vi "genImageMatrix.vi"(6 "Orientation":bool, 8 "Phase":dbl, 9 "Cycles":dbl, 10 "Y resolution":i32, 11 "X Resolution":i32) -> (1 "genSize":i32[](array[numeric]), 3 "Scan Image":u8[][](array[numeric]))   [LabVIEW 2017]
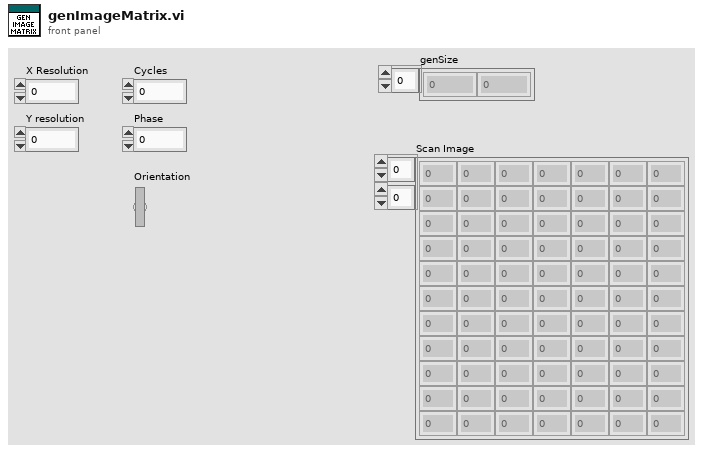
[diagram p1: front panel]
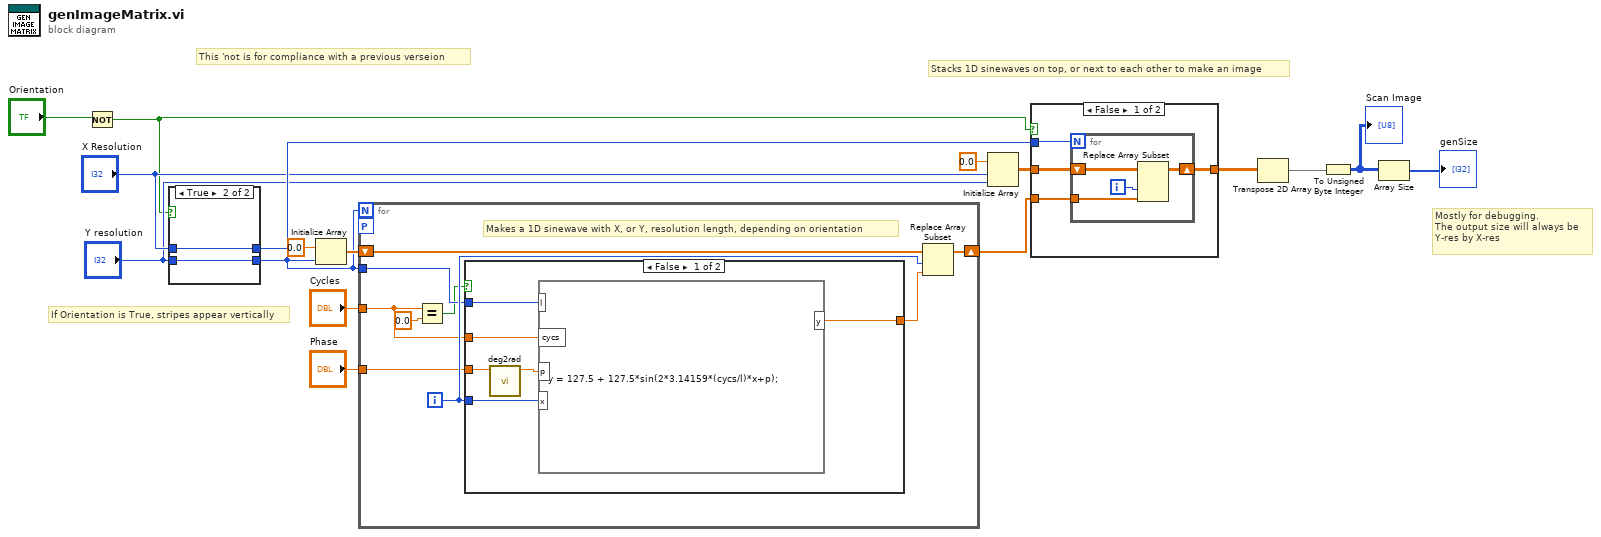
[diagram p0: block diagram]
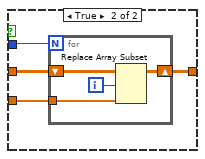
[diagram p2: hidden frame]
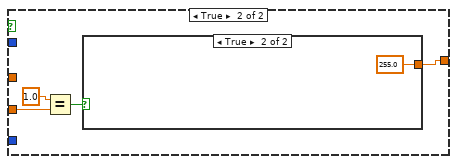
[diagram p4: hidden frame]
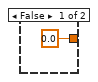
[diagram p5: hidden frame]
diagram:
  # "This 'not is for compliance with a previous verseion"
  # "Mostly for debugging.\nThe output size will always be\nY-res by X-res"
  # "Stacks 1D sinewaves on top, or next to each other to make an image"
  # "If Orientation is True, stripes appear vertically"
  n1 = Not(x="Orientation") -> (.not. x?=w1:bool)
  n2 = case shown="True" w1 {
    tunnel: [w18 w20] -> w9
    tunnel: "Y resolution" -> [w19 w20]
    tunnel: "X Resolution" -> [w18 w21]
    tunnel: [w19 w21] -> w7
    frame False {
    }
    frame True {
    }
  }
  n3 = Initialize Array(0.0 ("element"), w9) -> (w15:dbl[])
  n4 = for {
    N: w9 -> [_]
    shift-right: [w28] -> w8
    shift-left: w15 -> [w29]
    tunnel: "Cycles" -> [w22]
    tunnel: "Phase" -> [w26]
    tunnel: w9 -> [w25]
    workers-P: _ -> [_]
    i -> [w27]
    # "Makes a 1D sinewave with X, or Y, resolution length, depending on orientation"
    n5 = Equal?(x=w22, y=0.0) -> (x = y?=w24:bool)
    n6 = case shown="False" w24 {
      tunnel: [w36 w37] -> w30
      tunnel: w27 -> [w35 _]
      tunnel: w22 -> [w34 _]
      tunnel: w26 -> [w32 w40]
      tunnel: w25 -> [w33 _]
      frame False {
        n7 = call "deg2rad.vi"("Degrees"=w32) -> ("Radians"=w31:dbl)  [unwired: 10 in]
        n8 = formula code="y = 127.5 + 127.5*sin(2*3.14159*(cycs/l)*x+p);"("l"=w33, "cycs"=w34, "p"=w31, "x"=w35) -> ("y"=w36:dbl)
      }
      frame True {
        n9 = Equal?(x=1.0, y=w40) -> (x = y?=w38:bool)
        n10 = case shown="True" w38 {
          tunnel: [0.0 255.0] -> w37
          frame False {
          }
          frame True {
          }
        }
      }
    }
    n11 = Replace Array Subset(array=w29, new element=w30, index=w27) -> (w28:dbl[])
  }
  n12 = Initialize Array(0.0 ("element"), "X Resolution", "Y resolution") -> (w14:dbl[][])
  n13 = case shown="False" w1 {
    tunnel: w14 -> [w45 w54]
    tunnel: w8 -> [w44 w53]
    tunnel: [w43 w52] -> w4
    tunnel: w7 -> [w46 w51]
    frame False {
      n14 = for {
        N: w46 -> [_]
        shift-right: [w49] -> w43
        shift-left: w45 -> [w50]
        tunnel: w44 -> [w47]
        i -> [w48]
        n15 = Replace Array Subset(array=w50, new element=w47, index (col)=w48) -> (w49:dbl[][])  [unwired: 1 in]
      }
    }
    frame True {
      n16 = for {
        N: w51 -> [_]
        shift-right: [w55] -> w52
        shift-left: w54 -> [w58]
        tunnel: w53 -> [w56]
        i -> [w57]
        n17 = Replace Array Subset(array=w58, new element=w56, index (row)=w57) -> (w55:dbl[][])  [unwired: 1 in]
      }
    }
  }
  n18 = Transpose 2D Array(2D array=w4) -> (transposed array=w3:dbl[][])
  n19 = To Unsigned Byte Integer(number=w3) -> (unsigned 8bit integer=w11:u8[][])
  "Scan Image" <- w11
  n20 = Array Size(array=w11) -> (size(s)=→"genSize":i32[])
